vi "save configuration.vi"(8 "error in (no error)":errorcluster, 10 "Path":path, 11 "Camera":T1) -> (0 "error out":errorcluster, 3 "Camera out":T1)   [LabVIEW 2022 SP3, in "Vision.lvlib"]
uses:
  Vision.lvlib
  camera.ctl
  camera driver.ctl
  <vilib>/userDefined/High Color/IMAQdx.ctl
  C:/Users/Caleb/Desktop/nebraska-silicon-lab/pixel-gantry-control/Gantry/Shared Components/bin/uEyeDotNet.dll
  bin/uEyeDotNet.dll
  <vilib>/vision/driver/NI_Vision_Acquisition_Software.lvlib
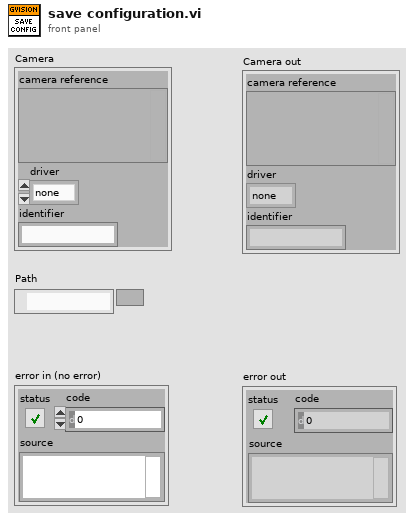
[diagram p1: front panel]
types:
  T1 = typedef "Vision.lvlib/camera.ctl" = cluster{"camera reference":variant, "driver":T2, "identifier":string}
  T2 = typedef "Vision.lvlib/camera driver.ctl" = enum16{"none", "ueye", "wmf", "imaqdx"}
  T3 = typedef "IMAQdx.ctl" = refnum<k21>
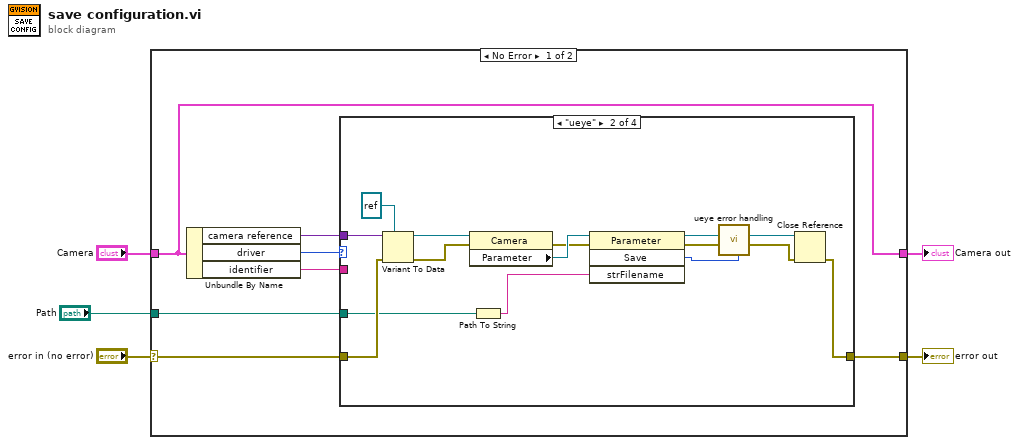
[diagram p0: block diagram]
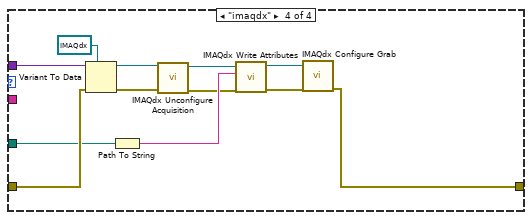
[diagram p4: hidden frame]
diagram:
  n1 = case shown="No Error" "error in (no error)" {
    selector: "error in (no error)" -> [w7 w42]
    tunnel: [w9 w42] -> w4
    tunnel: "Camera" -> [w8 w41]
    tunnel: [w8 w41] -> w2
    tunnel: "Path" -> [w6 _]
    frame No Error {
      n2 = Unbundle By Name(w8) -> ("camera reference"=w11:variant, "driver"=w12:T2, "identifier"=w10:string)
      n3 = case shown="\"ueye\"" w12 {
        tunnel: w11 -> [_ w27 _ w40]
        tunnel: w10 -> [_ _ _ _]
        tunnel: w7 -> [w13 w24 w28 w38]
        tunnel: [w13 w16 w28 w29] -> w9
        tunnel: w6 -> [_ w20 _ w37]
        frame "none" {
        }
        frame "ueye" {
          n4 = Variant To Data(error in=w24, type=refnum<k24> refnum ("reference"), Variant=w27) -> (data=w25:refnum<k24>, error out=w23:errorcluster)
          n5 = property class="Camera"(reference=w25, error in=w23) -> (error out=w21:errorcluster, "Parameter"=w22:refnum<k24>)  [unwired: 1 out]
          n6 = Path To String(path=w20) -> (string=w19:string)
          n7 = invoke class="Parameter" method="Save"(reference=w22, error in=w21, "strFilename"=w19) -> (reference out=w14:refnum<k24>, error out=w18:errorcluster, "Save"=w15:i32)  [unwired: 1 in, 1 out]
          n8 = call "ueye error handling.vi"("Error Code"=w15, "reference in"=w14, "Error In"=w18) -> ("Error Out"=w17:errorcluster)  [unwired: 8 in]
          n9 = Close Reference(reference=w14, error in (no error)=w17) -> (error out=w16:errorcluster)
        }
        frame "wmf" {
        }
        frame "imaqdx" {
          n10 = Variant To Data(error in=w38, type=T3 refnum ("Session In"), Variant=w40) -> (data=w33:T3, error out=w35:errorcluster)
          n11 = Path To String(path=w37) -> (string=w36:string)
          n12 = call <vilib>:"IMAQdx Unconfigure Acquisition.vi"("error in"=w35, "Session In"=w33) -> ("error out"=w34:errorcluster, "Session Out"=w32:T3)  [unwired: 8 in]
          n13 = call <vilib>:"IMAQdx Write Attributes.vi"("error in"=w34, "Filename"=w36, "Session In"=w32) -> ("error out"=w30:errorcluster, "Session Out"=w31:T3)  [unwired: 7 in]
          n14 = call <vilib>:"IMAQdx Configure Grab.vi"("error in"=w30, "Session In"=w31) -> ("error out"=w29:errorcluster)  [unwired: 8 in, 1 out]
        }
      }
    }
    frame Error {
    }
  }
  "error out" <- w4
  "Camera out" <- w2
